vi "Pre-Build Custom Action.vi"(10 "Variant":variant) -> (0 "error out":errorcluster)   [LabVIEW 2013]
uses:
  pre-build properties -- cluster.ctl
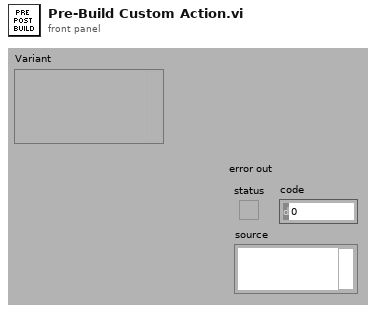
[diagram p1: front panel]
types:
  T1 = typedef "pre-build properties -- cluster.ctl" = cluster{"Output Package File Path":path, "Package Member Source Files":path[], "Passwords":string[], "Product Name":string, "Package Version":string, "Package LabVIEW Version":string, "Package Source Folder":path, "Package Name":string, "Build Failure":bool}
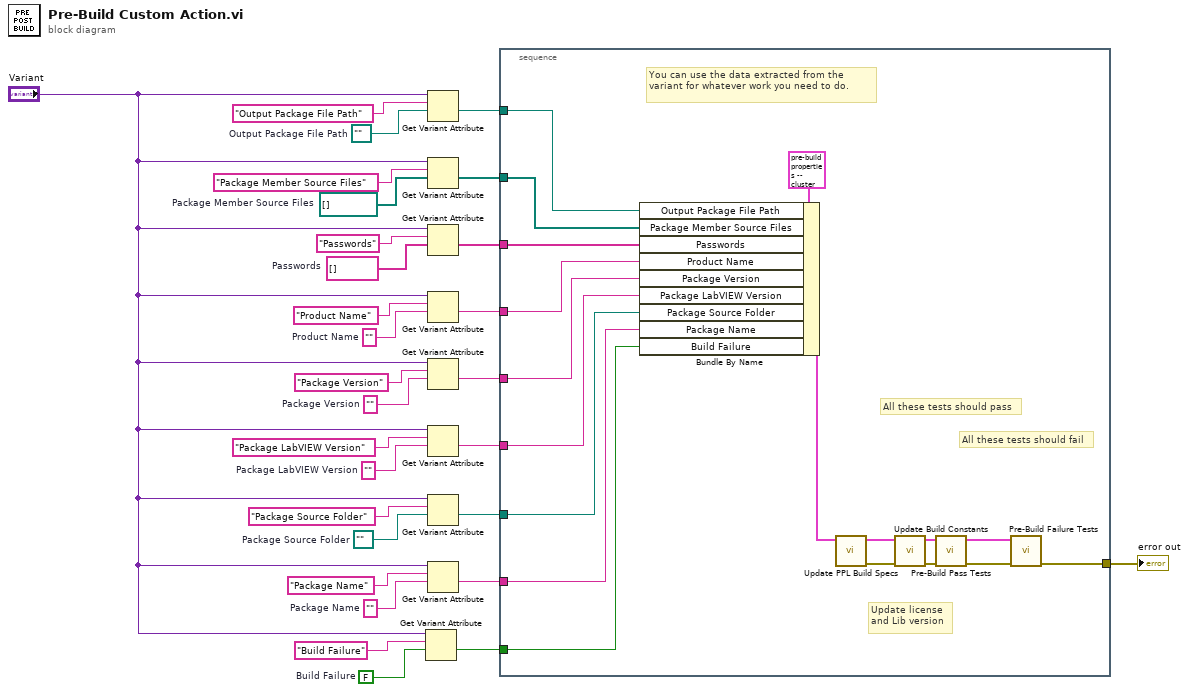
[diagram p0: block diagram]
diagram:
  w4 = FALSE  # Build Failure
  w14 = path ""  # Package Source Folder
  w15 = ""  # Package Name
  w18 = ""  # Package LabVIEW Version
  w20 = ""  # Package Version
  w22 = ""  # Product Name
  w24 = string[] []  # Passwords
  w26 = path[] []  # Package Member Source Files
  w28 = path ""  # Output Package File Path
  n1 = Get Variant Attribute(Variant="Variant", name="Build Failure", default value (empty Variant)=w4) -> (value=w2:bool)  [unwired: 1 in, 3 out]
  n2 = Get Variant Attribute(Variant="Variant", name="Output Package File Path", default value (empty Variant)=w28) -> (value=w13:path)  [unwired: 1 in, 3 out]
  n3 = Get Variant Attribute(Variant="Variant", name="Package Member Source Files", default value (empty Variant)=w26) -> (value=w12:path[])  [unwired: 1 in, 3 out]
  n4 = Get Variant Attribute(Variant="Variant", name="Passwords", default value (empty Variant)=w24) -> (value=w11:string[])  [unwired: 1 in, 3 out]
  n5 = Get Variant Attribute(Variant="Variant", name="Product Name", default value (empty Variant)=w22) -> (value=w10:string)  [unwired: 1 in, 3 out]
  n6 = Get Variant Attribute(Variant="Variant", name="Package Version", default value (empty Variant)=w20) -> (value=w9:string)  [unwired: 1 in, 3 out]
  n7 = Get Variant Attribute(Variant="Variant", name="Package LabVIEW Version", default value (empty Variant)=w18) -> (value=w8:string)  [unwired: 1 in, 3 out]
  n8 = Get Variant Attribute(Variant="Variant", name="Package Source Folder", default value (empty Variant)=w14) -> (value=w7:path)  [unwired: 1 in, 3 out]
  n9 = Get Variant Attribute(Variant="Variant", name="Package Name", default value (empty Variant)=w15) -> (value=w6:string)  [unwired: 1 in, 3 out]
  n10 = stacked-sequence {
    tunnel: w13 -> [w46]
    tunnel: w12 -> [w45]
    tunnel: w11 -> [w44]
    tunnel: w10 -> [w43]
    tunnel: w9 -> [w42]
    tunnel: w8 -> [w41]
    tunnel: w7 -> [w38]
    tunnel: w6 -> [w40]
    tunnel: w2 -> [w39]
    tunnel: [w33] -> w1
    frame #0 {
      # "Update license\nand Lib version"
      # "All these tests should fail"
      # "All these tests should pass"
      # "You can use the data extracted from the variant for whatever work you need to do."
      n11 = Bundle By Name(cluster=T1 {"Output Package File Path"=path "", "Package Member Source Files"=[], "Passwords"=[], "Product Name"="", "Package Version"="", "Package LabVIEW Version"="", "Package Source Folder"=path "", "Package Name"="", "Build Failure"=FALSE}, "Output Package File Path"=w46, "Package Member Source Files"=w45, "Passwords"=w44, "Product Name"=w43, "Package Version"=w42, "Package LabVIEW Version"=w41, "Package Source Folder"=w38, "Package Name"=w40, "Build Failure"=w39) -> (w32:T1)
      n12 = call "Update PPL Build Specs.vi"("Pre-Build Properties"=w32) -> ("error out"=w30:errorcluster, "Pre-Build Properties dup"=w31:T1)  [unwired: 9 in]
      n13 = call "Update Build Constants.vi"("error in (no error)"=w30, "Pre-Build Properties"=w31) -> ("error out"=w34:errorcluster, "Pre-Build Properties dup"=w35:T1)  [unwired: 8 in]
      n14 = call "Pre-Build Pass Tests.vi"("error in (no error)"=w34, "Pre-Build Properties"=w35) -> ("error out"=w36:errorcluster, "Pre-Build Properties dup"=w37:T1)  [unwired: 8 in]
      n15 = call "Pre-Build Failure Tests.vi"("error in (no error)"=w36, "Pre-Build Properties"=w37) -> ("error out"=w33:errorcluster)  [unwired: 8 in, 1 out]
    }
  }
  "error out" <- w1
